vi "Nonlinear Curve Fit LM.vi"(0 "Y":dbl[](array[numeric]), 1 "f(x,a)":T1, 2 "data":variant, 5 "X":dbl[](array[numeric]), 7 "Weight":dbl[](array[numeric]), 9 "initial parameters":dbl[](array[numeric]), 11 "error in (no error)":errorcluster, 12 "termination":cluster{"max iteration":i32, "tolerance":dbl}={"max iteration"=200, "tolerance"=1e-08}) -> (3 "number of function calls":i32, 4 "best nonlinear fit":dbl[](array[numeric]), 6 "best fit parameters":dbl[](array[numeric]), 8 "covariance":T2, 14 "residue":dbl, 15 "error out":errorcluster)   [LabVIEW 2010, in "NI_Gmath.lvlib"]
doc: "Uses the Levenberg-Marquardt algorithm to determine the set of parameters that best fit the set of input data points (<B>X</B>, <B>Y</B>) as expressed by a nonlinear function y = <B>f(x,a)</B>, where a is the set of parameters. You must manually select the polymorphic instance to use."
uses:
  NI_Gmath.lvlib
  RealMatrix.ctl
  LM model function reference.ctl
  stopping criteria.ctl
  LM model function.ctl
  LM_output select.ctl
  Real Inverse Matrix.vi
  NI_AALBase.lvlib
  NI_Matrix.lvlib
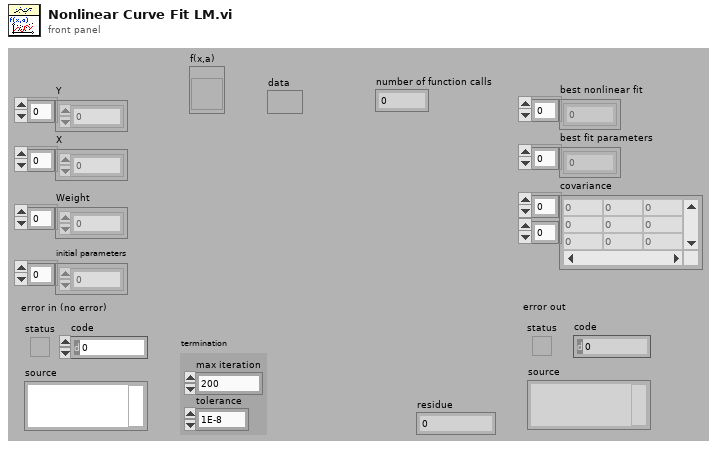
[diagram p1: front panel]
types:
  T1 = typedef "NI_Gmath.lvlib/LM model function reference.ctl" = refnum<vi>
  T2 = typedef "NI_Matrix.lvlib/RealMatrix.ctl" = dbl[][]
  T3 = typedef "NI_Gmath.lvlib/LM model function.ctl" = cluster{"f(x,a)":T1, "data":variant}
  T4 = typedef "NI_Gmath.lvlib/stopping criteria.ctl" = cluster{"function tolerance":dbl, "parameter tolerance":dbl, "max iterations":i32, "max function calls":i32, "gradient tolerance":dbl, "max time (sec)":dbl}
  T5 = typedef "NI_Gmath.lvlib/stopping criteria with time.ctl" = cluster{"function tolerance":dbl, "parameter tolerance":dbl, "max iterations":i32, "max function calls":i32, "gradient tolerance":dbl, "max time (sec)":dbl, "initial tick count":u32}
  T6 = typedef "NI_Gmath.lvlib/LM_output select.ctl" = cluster{"model function":bool, "gradient":bool}
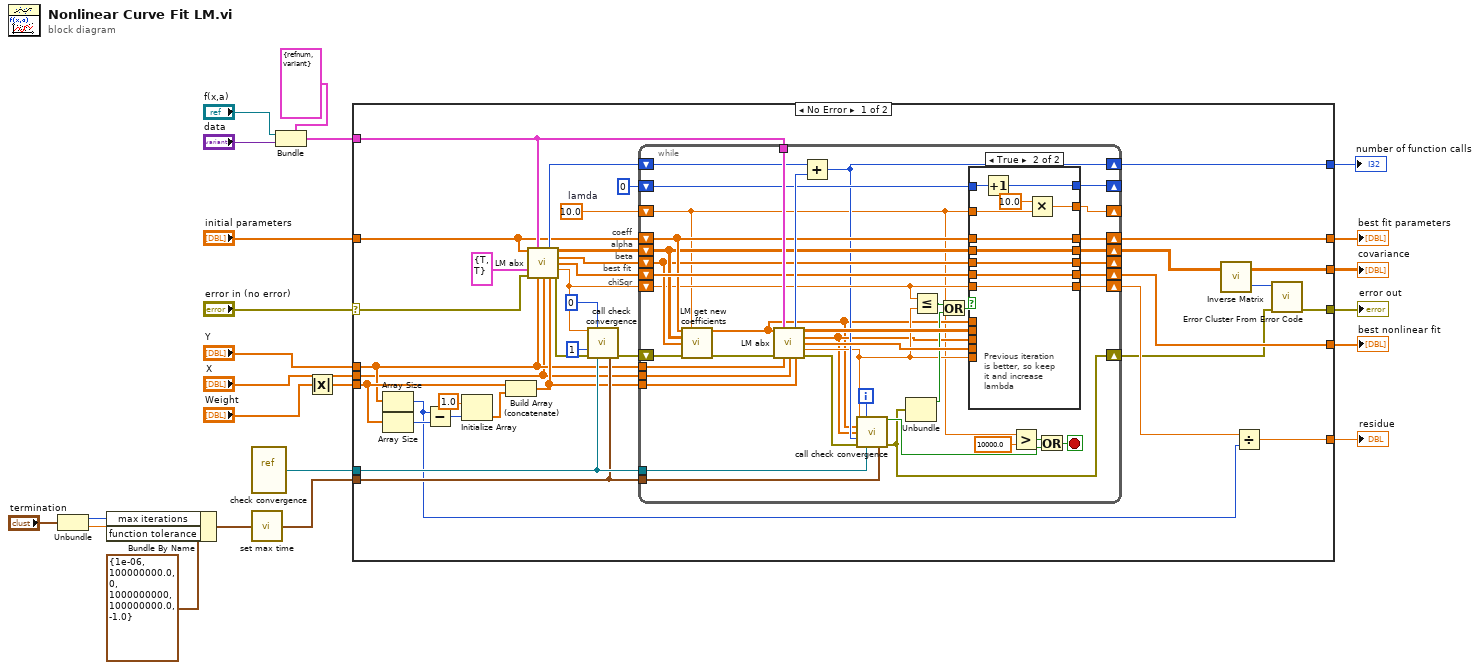
[diagram p0: block diagram]
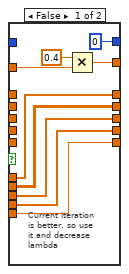
[diagram p2: hidden frame]
diagram:
  n1 = Unbundle("termination") -> ("max iteration"=w11:i32, "tolerance"=w10:dbl)
  n2 = Bundle By Name(cluster=T4 {"function tolerance"=1e-06, "parameter tolerance"=100000000.0, "max iterations"=0, "max function calls"=1000000000, "gradient tolerance"=100000000.0, "max time (sec)"=-1.0} ("stopping criteria"), "max iterations"=w11, "function tolerance"=w10) -> (w3:T4)
  n3 = vi-ref "check convergence.vi"() -> (w9:refnum<vi>)
  n4 = call "set max time.vi"("stopping criteria"=w3) -> ("stopping criteria"=w2:T5)
  n5 = Bundle(cluster=T3 {"f(x,a)"=refnum, "data"=variant} ("model function"), "f(x,a)"="f(x,a)", "data"="data") -> (w5:T3)
  n6 = Absolute Value(x="Weight") -> (abs(x)=w1:dbl[])
  n7 = case shown="No Error" "error in (no error)" {
    selector: "error in (no error)" -> [w38 w119]
    tunnel: [w25 _] -> w23
    tunnel: [w53 _] -> w22
    tunnel: "initial parameters" -> [w29 _]
    tunnel: [w34 _] -> w20
    tunnel: [w51 _] -> w19
    tunnel: w1 -> [w47 _]
    tunnel: "Y" -> [w43 _]
    tunnel: w2 -> [w58 _]
    tunnel: "X" -> [w36 _]
    tunnel: [w45 w119] -> w15
    tunnel: w5 -> [w37 _]
    tunnel: w9 -> [w59 _]
    tunnel: [w27 _] -> w8
    frame No Error {
      w55 = 10.0  # lamda
      # "best fit"
      # "chiSqr"
      # "beta"
      # "alpha"
      # "coeff"
      n8 = Array Size(array=w43) -> (size(s)=w24:i32)
      n9 = Array Size(array=w47) -> (size(s)=w50:i32)
      n10 = Subtract(x=w24, y=w50) -> (x-y=w49:i32)
      n11 = Initialize Array(1.0, w49) -> (w48:dbl[])
      n12 = Build Array (concatenate)(w47, w48) -> (w57:dbl[])
      n13 = call "LM abx.vi"("coefficients"=w29, "model function"=w37, "output control"=T6 {"model function"=TRUE, "gradient"=TRUE}, "error in (no error)"=w38, "Y"=w43, "X"=w36, "Weight"=w57) -> ("number of function calls"=w39:i32, "alpha"=w56:T2, "beta"=w44:dbl[], "best fit"=w35:dbl[], "chiSqr"=w42:dbl, "error out"=w41:errorcluster)  [unwired: 3 in]
      n14 = call "call check convergence.vi"("f"=w42, "current iteration"=0, "number of function evaluations"=1, "error in"=w41, "vi reference"=w59, "stopping criteria"=w58) -> ("error out"=w40:errorcluster)  [unwired: 5 in, 4 out]
      n15 = while {
        tunnel: w36 -> [w91]
        tunnel: w43 -> [w92]
        tunnel: w57 -> [w90]
        shift-left: w42 -> [w80]
        shift-right: [w79] -> w54
        shift-left: w44 -> [w81]
        shift-right: [w97] -> _
        shift-left: w56 -> [w82]
        shift-right: [w98] -> w30
        shift-left: w29 -> [w83]
        shift-right: [w94] -> w25
        shift-left: w55 -> [w65]
        shift-right: [w93] -> _
        shift-right: [w60] -> w33
        shift-left: w40 -> [w96]
        tunnel: w37 -> [w89]
        tunnel: w59 -> [w68]
        tunnel: w58 -> [w67]
        shift-right: [w71] -> w27
        shift-left: w39 -> [w87]
        shift-right: [w84] -> w34
        shift-left: w35 -> [w86]
        shift-right: [w74] -> _
        shift-left: 0 -> [w75]
        i -> [w72]
        stop <- w61 stop-if-true
        n16 = call "LM get new coefficients.vi"("Coefficients"=w83, "lamda"=w65, "Alpha"=w82, "Beta"=w81, "error in (no error)"=w96) -> ("New Coefficients"=w66:dbl[], "error out"=w95:errorcluster)  [unwired: 9 in]
        n17 = call "LM abx.vi"("coefficients"=w66, "model function"=w89, "error in (no error)"=w95, "Y"=w92, "X"=w91, "Weight"=w90) -> ("number of function calls"=w99:i32, "alpha"=w88:T2, "beta"=w69:dbl[], "best fit"=w85:dbl[], "chiSqr"=w70:dbl, "error out"=w73:errorcluster)  [unwired: 4 in]
        n18 = Add(x=w87, y=w99) -> (x+y=w71:i32)
        n19 = call "call check convergence.vi"("f"=w70, "current iteration"=w72, "X"=w66, "gradient"=w69, "number of function evaluations"=w71, "error in"=w73, "vi reference"=w68, "stopping criteria"=w67) -> ("stop?"=w63:bool, "error out"=w60:errorcluster)  [unwired: 3 in, 3 out]
        n20 = Unbundle(w60) -> ("status"=w77:bool)  [unwired: 2 out]
        n21 = Less Or Equal?(x=w80, y=w70) -> (x <= y?=w78:bool)
        n22 = Or(x=w78, y=w77) -> (x .or. y?=w76:bool)
        n23 = case shown="True" w76 {
          tunnel: [w105 w118] -> w98
          tunnel: w82 -> [_ w118]
          tunnel: [w104 w117] -> w97
          tunnel: w66 -> [w101 _]
          tunnel: w81 -> [_ w117]
          tunnel: w83 -> [_ w116]
          tunnel: [w101 w116] -> w94
          tunnel: [w106 w112] -> w93
          tunnel: w80 -> [_ w115]
          tunnel: w70 -> [w102 _]
          tunnel: [w102 w115] -> w79
          tunnel: w65 -> [w108 w113]
          tunnel: w88 -> [w105 _]
          tunnel: w69 -> [w104 _]
          tunnel: w86 -> [_ w111]
          tunnel: w85 -> [w103 _]
          tunnel: [w103 w111] -> w84
          tunnel: w75 -> [_ w110]
          tunnel: [0 w109] -> w74
          frame False {
            # "Current iteration\nis better, so use\nit and decrease \nlambda"
            n24 = Multiply(x=0.4, y=w108) -> (x*y=w106:dbl)
          }
          frame True {
            # "Previous iteration\nis better, so keep\nit and increase \nlambda"
            n25 = Increment(x=w110) -> (x+1=w109:i32)
            n26 = Multiply(x=10.0, y=w113) -> (x*y=w112:dbl)
          }
        }
        n27 = Greater?(x=w65, y=10000.0) -> (0:w62:bool)
        n28 = Or(x=w62, y=w63) -> (x .or. y?=w61:bool)
      }
      n29 = call-poly "Inverse Matrix.vi"("Input Matrix"=w30) -> ("error"=w46:i32, "Inverse Matrix"=w51:T2)  [unwired: 1 in]
      n30 = Divide(x=w54, y=w24) -> (x/y=w53:dbl)
      n31 = call "Error Cluster From Error Code.vi"("error in (no error)"=w33, "error code (0)"=w46) -> ("error out"=w45:errorcluster)  [unwired: 7 in]
    }
    frame Error {
    }
  }
  "residue" <- w22
  "best fit parameters" <- w23
  "best nonlinear fit" <- w20
  "error out" <- w15
  "covariance" <- w19
  "number of function calls" <- w8
